vi "AutoTrackRobot.vi"(11 "StartCoordinates":dbl[](array[numeric])) -> (3 "Coordinates":dbl[](array[numeric]))   [LabVIEW 2018]
uses:
  Globals.vi
  navx-mxp/labview/navX Library v2/navX Library v2.lvlib
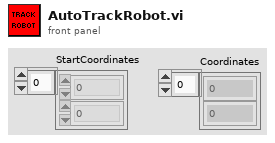
[diagram p1: front panel]
types:
  T1 = typedef "navX Library v2.lvlib/Z900_navX_DeviceTypeDef.ctl" = cluster{"Interface":cluster{"Protocol":T2, "Update Rate (4Hz-100Hz)":u8, "navX Open TypeDef":variant}, "Notify Packet":refnum<notifier>, "Loop VI Refnum":refnum<vi>, "Ready to Close Occurrence Refnum":refnum<k4>}
  T2 = typedef "navX Library v2.lvlib/Z900_navX_ProtocolTypeDef.ctl" = enum16{"SERIAL", "I2C", "SPI"}
  T3 = cluster{"Velocity X":dbl, "Velocity Y":dbl, "Velocity Z":dbl, "Displacement X":dbl, "Displacement Y":dbl, "Displacement Z":dbl}
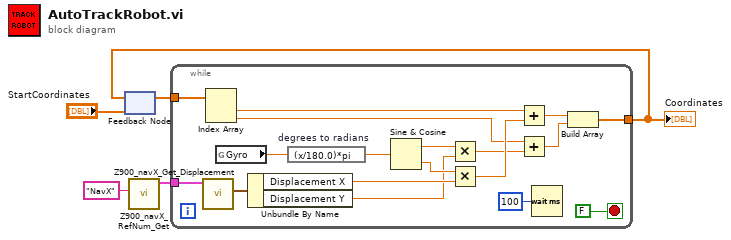
[diagram p0: block diagram]
diagram:
  n1 = feedback #1("StartCoordinates") -> (w5:dbl[])
  n2 = call "Z900_navX_RefNum_Get.vi"("refnum name"="NavX") -> ("navX Device"=w1:T1)  [unwired: 9 in, 1 out]
  n3 = while {
    tunnel: w5 -> [w21]
    tunnel: [w12] -> w3
    tunnel: w1 -> [w6]
    stop <- FALSE stop-if-true
    n4 = call "Z900_navX_Get_Displacement.vi"("navX Device"=w6) -> ("Displacement"=w7:T3)  [unwired: 7 in, 3 out]
    n5 = Index Array(array=w21) -> (element #1=w20:dbl, element #2=w16:dbl)  [unwired: 2 in]
    n6 = global read "Globals.vi" "Gyro"() -> (w22:dbl)
    n7 = Unbundle By Name(w7) -> ("Displacement X"=w9:dbl, "Displacement Y"=w8:dbl)
    n8 = expression code="(x/180.0)*pi" "degrees to radians"(w22) -> (w10:dbl)
    n9 = Sine & Cosine(0:w10) -> (1:w19:dbl, 2:w18:dbl)
    n10 = Multiply(x=w19, y=w8) -> (x*y=w15:dbl)
    n11 = Multiply(x=w18, y=w9) -> (x*y=w17:dbl)
    n12 = Add(x=w20, y=w17) -> (x+y=w14:dbl)
    n13 = Add(x=w16, y=w15) -> (x+y=w13:dbl)
    n14 = Wait (ms)(milliseconds to wait=u32 100) -> ()  [unwired: 1 out]
    n15 = Build Array(w14, w13) -> (w12:dbl[])
  }
  "Coordinates" <- w3
  n16 = feedback-in #1(w3) -> ()
